vi "fpga_counter.vi"(7 "max counts":i16, 10 "reset? (F)":bool, 11 "count? (T)":bool=TRUE) -> (0 "completed? (switch)":bool, 3 "completed?":bool)   [LabVIEW 2021]
doc: "Simple counter."
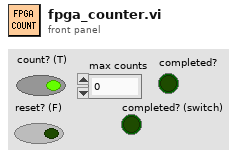
[diagram p1: front panel]
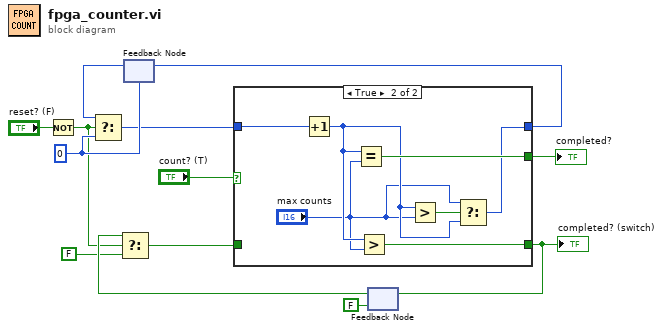
[diagram p0: block diagram]
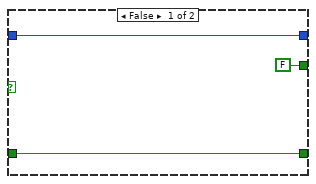
[diagram p2: hidden frame]
diagram:
  w12 = i16 0 ("max counts")
  n1 = Not(x="reset? (F)") -> (.not. x?=w1:bool)
  n2 = feedback #1(w12) -> (w11:i16)
  n3 = Select(t=w11, s=w1, f=w12) -> (s? t:f=w10:i16)
  n4 = feedback #2(FALSE) -> (w4:bool)
  n5 = Select(t=w4, s=w1, f=FALSE) -> (s? t:f=w3:bool)
  n6 = case shown="True" "count? (T)" {
    tunnel: w10 -> [w16 w23]
    tunnel: [FALSE w22] -> w9
    tunnel: [w16 w20] -> w7
    tunnel: [w14 w19] -> w6
    tunnel: w3 -> [w14 _]
    frame False {
    }
    frame True {
      n7 = Increment(x=w23) -> (x+1=w18:i16)
      n8 = Equal?(x=w18, y="max counts") -> (x = y?=w22:bool)
      n9 = Greater?(x=w18, y="max counts") -> (0:w19:bool)
      n10 = Greater?(x=w18, y="max counts") -> (0:w21:bool)
      n11 = Select(t="max counts", s=w21, f=w18) -> (s? t:f=w20:i16)
    }
  }
  "completed?" <- w9
  "completed? (switch)" <- w6
  n12 = feedback-in #1(w7) -> ()
  n13 = feedback-in #2(w6) -> ()
